vi "configureOutput.vi"(6 "sofwareTrigger?":bool, 8 "error in (no error)":errorcluster, 9 "Data":variant, 10 "Config":T1, 11 "SpinCore in":refnum<class "SpinCore.lvclass">) -> (0 "error out":errorcluster, 3 "SpinCore out":refnum<class "SpinCore.lvclass">)   [LabVIEW 2011, in "Hardware.lvlib" / "Channels.lvlib" / "SpinCore.lvclass"]
doc: "Data is a varient cluster. \n\nThe varient is transformed into the correct cluster, and that cluster is stored.\n(Not Implemented for Ramp function)"
uses:
  SpinCore.lvclass
  Generic/DDSOutput.lvclass
  SpinCore.lvclass/SpinCore.ctl
panel:
  out "Data":dbl
  out "load time":dbl
  out "data (time, freq, amplitude, phase)":dbl[][](array[numeric]) format="%#.7g"
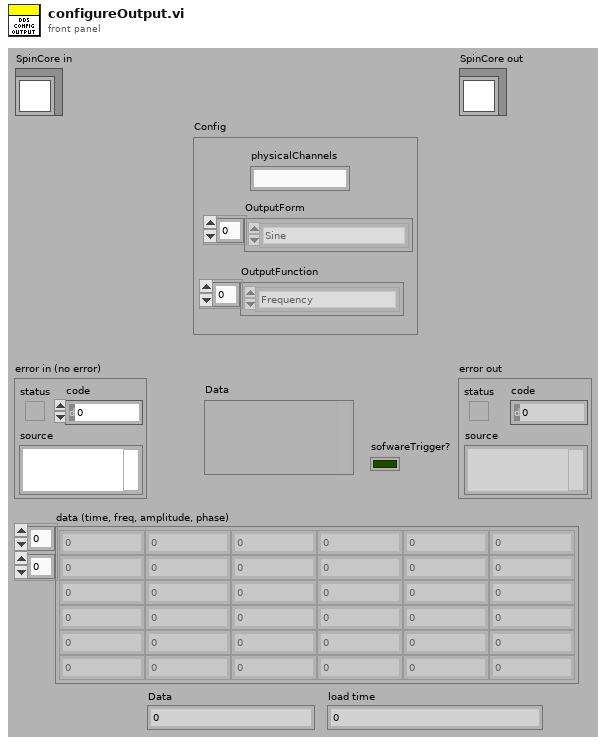
[diagram p1: front panel]
types:
  T1 = cluster{"OutputForm":enum16{"Sine", "Square", "Triangle", "Arbitrary"}[], "OutputFunction":enum16{"Frequency", "Ramp", "Sequence"}[], "physicalChannels":string}
  T2 = cluster{"Frequency(MHz)":dbl, "Amplitude":dbl, "Phase":dbl, "OutputForm":enum16{"Sine", "Square", "Triangle", "Arbitrary"}}[]
  T3 = cluster{"data (time, freq, amplitude, phase)":dbl[][]}
  T4 = cluster{"data (time, freq, amplitude, phase)":dbl[][]}[]
  T5 = cluster{"Frequency(MHz)":dbl, "Amplitude":dbl, "Phase":dbl, "OutputForm":enum16{"Sine", "Square", "Triangle", "Arbitrary"}}
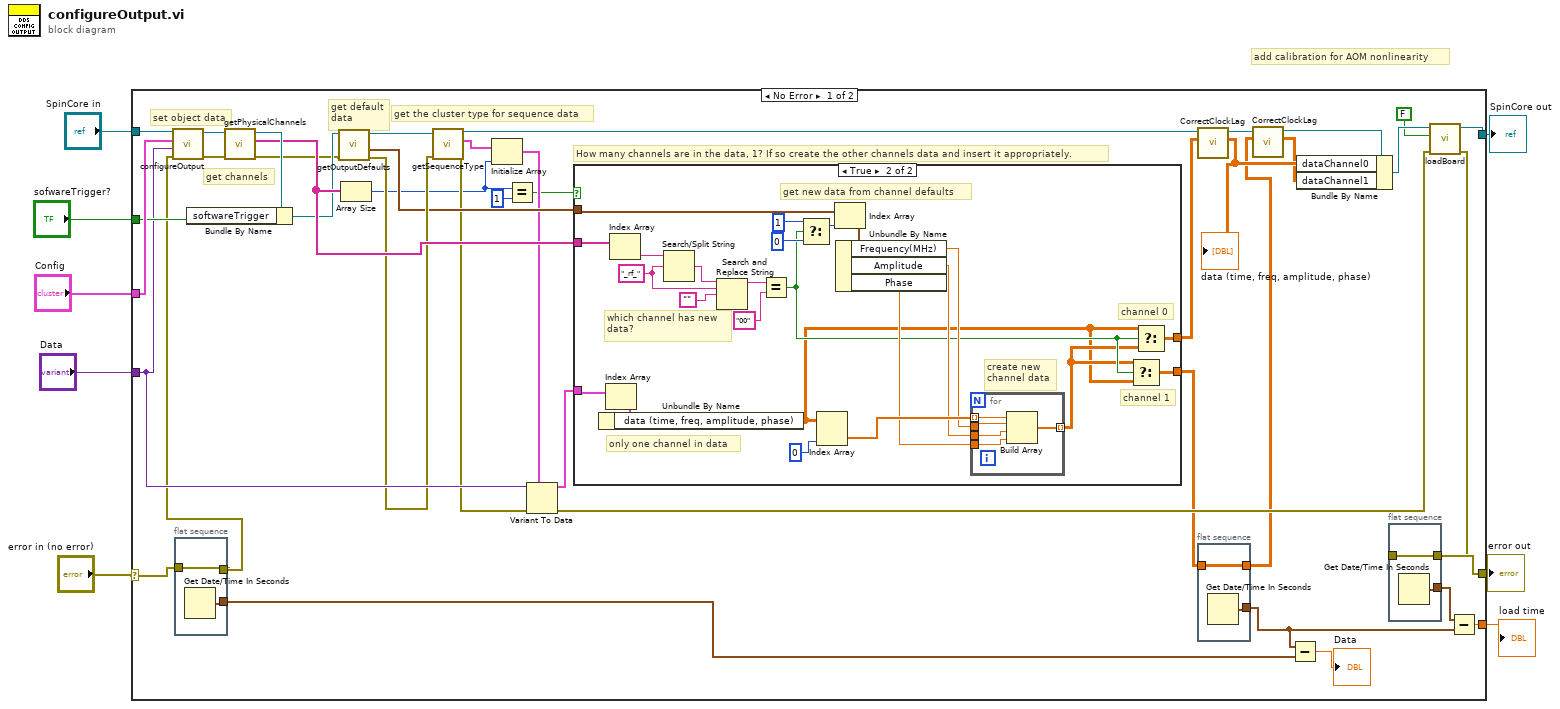
[diagram p0: block diagram]
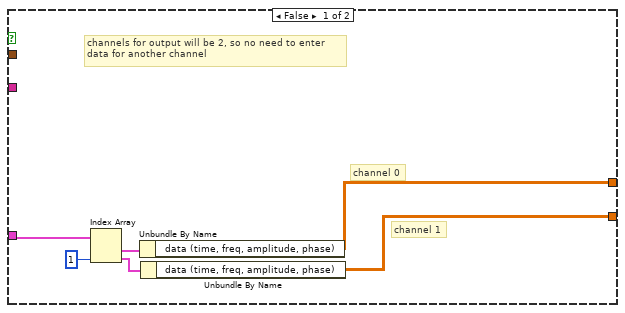
[diagram p2: hidden frame]
diagram:
  # "add calibration for AOM nonlinearity"
  n1 = case shown="No Error" "error in (no error)" {
    selector: "error in (no error)" -> [w22 w91]
    tunnel: [w26 w91] -> w8
    tunnel: [w46 w92] -> w7
    tunnel: "SpinCore in" -> [w49 w92]
    tunnel: "Config" -> [w48 _]
    tunnel: "Data" -> [w40 _]
    tunnel: "sofwareTrigger?" -> [w45 _]
    tunnel: [w23 _] -> w1
    frame No Error {
      # "get default\ndata"
      # "get channels"
      # "set object data"
      # "get the cluster type for sequence data"
      # "How many channels are in the data, 1? If so create the other channels data and insert it appropriately."
      n2 = call-parent "configureOutput.vi"("error in (no error)"=w21, "Data"=w40, "Config"=w48, "DDSOutput in"=w49) -> ("error out"=w44:errorcluster, "DDSOutput out"=w43:refnum<class "SpinCore.lvclass">)  [unwired: 6 in]
      n3 = flat-sequence {
        tunnel: [w51] -> w21
        tunnel: w22 -> [w51]
        tunnel: [w50] -> w17
        frame #0 {
          n4 = Get Date/Time In Seconds() -> (seconds since 1Jan1904=w50:timestamp)
        }
      }
      n5 = call "getPhysicalChannels.vi"("error in (no error)"=w44, "DDSOutput in"=w43) -> ("error out"=w36:errorcluster, "physicalChannels"=w41:string[], "DDSOutput out"=w42:refnum<class "SpinCore.lvclass">)  [unwired: 7 in]
      n6 = Bundle By Name(cluster=w42, "softwareTrigger"=w45) -> (w37:refnum<class "SpinCore.lvclass">)
      n7 = call "getOutputDefaults.vi"("error in (no error)"=w36, "DDSOutput in"=w37) -> ("error out"=w35:errorcluster, "Defaults"=w34:T2, "DDSOutput out"=w38:refnum<class "SpinCore.lvclass">)  [unwired: 6 in, 1 out]
      n8 = Array Size(array=w41) -> (size(s)=w29:i32)
      n9 = call "getSequenceType.vi"("error in (no error)"=w35, "DDSOutput in"=w38) -> ("error out"=w32:errorcluster, "Sequence"=w33:T3, "DDSOutput out"=w15:refnum<class "SpinCore.lvclass">)  [unwired: 7 in]
      n10 = Initialize Array(w33, w29) -> (w31:T4)
      n11 = Equal?(x=w29, y=1) -> (x = y?=w28:bool)
      n12 = Variant To Data(error in=w32, type=w31, Variant=w40) -> (data=w30:T4, error out=w20:errorcluster)
      n13 = case shown="True" w28 {
        tunnel: w41 -> [_ w81]
        tunnel: w34 -> [_ w74]
        tunnel: w30 -> [w61 w75]
        tunnel: [w59 w65] -> w14
        tunnel: [w57 w64] -> w19
        frame False {
          # "channel 1"
          # "channel 0"
          # "channels for output will be 2, so no need to enter\ndata for another channel"
          n14 = Index Array(array=w61, index #2=1) -> (element #1=w60:T3, element #2=w58:T3)  [unwired: 1 in]
          n15 = Unbundle By Name(w60) -> ("data (time, freq, amplitude, phase)"=w59:dbl[][])
          n16 = Unbundle By Name(w58) -> ("data (time, freq, amplitude, phase)"=w57:dbl[][])
        }
        frame True {
          w83 = "_rf_"
          # "get new data from channel defaults"
          # "only one channel in data"
          # "create new\nchannel data"
          # "channel 1"
          # "channel 0"
          # "which channel has new\ndata?"
          n17 = Index Array(array=w75) -> (element=w73:T3)  [unwired: 1 in]
          n18 = Unbundle By Name(w73) -> ("data (time, freq, amplitude, phase)"=w62:dbl[][])
          n19 = Index Array(array=w81) -> (element=w85:string)  [unwired: 1 in]
          n20 = Search/Split String(string=w85, search string/char (-)=w83) -> (match + rest of string=w84:string)  [unwired: 1 in, 2 out]
          n21 = Search and Replace String(input string=w84, search string=w83, replace string="") -> (result string=w79:string)  [unwired: 5 in, 3 out]
          n22 = Equal?(x=w79, y="00") -> (x = y?=w66:bool)
          n23 = Select(t=1, s=w66, f=0) -> (s? t:f=w78:i32)
          n24 = Index Array(array=w62, index (col)=0) -> (element=w70:dbl[])  [unwired: 1 in]
          n25 = Index Array(array=w74, index=w78) -> (element=w72:T5)
          n26 = Unbundle By Name(w72) -> ("Frequency(MHz)"=w69:dbl, "Amplitude"=w68:dbl, "Phase"=w67:dbl)
          n27 = for {
            tunnel: w70 -> [w90] mode=indexing
            tunnel: w69 -> [w89]
            tunnel: w68 -> [w88]
            tunnel: w67 -> [w87]
            tunnel: [w86] -> w63 mode=indexing
            n28 = Build Array(w90, w89, w88, w87) -> (w86:dbl[])
          }
          n29 = Select(t=w63, s=w66, f=w62) -> (s? t:f=w64:dbl[][])
          n30 = Select(t=w62, s=w66, f=w63) -> (s? t:f=w65:dbl[][])
        }
      }
      n31 = call "CorrectClockLag.vi"("data (time, freq, amplitude, phase)"=w14, "SpinCore in"=w15) -> ("data (time, freq, amplitude, phase)"=w13:dbl[][], "SpinCore out"=w12:refnum<class "SpinCore.lvclass">)  [unwired: 7 in, 1 out]
      "data (time, freq, amplitude, phase)" <- w13
      n32 = flat-sequence {
        tunnel: [w55] -> w18
        tunnel: [w54] -> w10
        tunnel: w19 -> [w54]
        frame #0 {
          n33 = Get Date/Time In Seconds() -> (seconds since 1Jan1904=w55:timestamp)
        }
      }
      n34 = call "CorrectClockLag.vi"("data (time, freq, amplitude, phase)"=w10, "SpinCore in"=w12) -> ("data (time, freq, amplitude, phase)"=w11:dbl[][], "SpinCore out"=w9:refnum<class "SpinCore.lvclass">)  [unwired: 7 in, 1 out]
      n35 = Subtract(x=w18, y=w17) -> (x-y=→"Data":dbl)
      n36 = Bundle By Name(cluster=w9, "dataChannel0"=w13, "dataChannel1"=w11) -> (w47:refnum<class "SpinCore.lvclass">)
      n37 = flat-sequence {
        tunnel: [w53] -> w24
        tunnel: [w52] -> w26
        tunnel: w25 -> [w52]
        frame #0 {
          n38 = Get Date/Time In Seconds() -> (seconds since 1Jan1904=w53:timestamp)
        }
      }
      n39 = call "loadBoard.vi"("error in (no error)"=w20, "continuous"=FALSE, "SpinCore in"=w47) -> ("error out"=w25:errorcluster, "SpinCore out"=w46:refnum<class "SpinCore.lvclass">)  [unwired: 7 in]
      n40 = Subtract(x=w24, y=w18) -> (x-y=w23:dbl)
    }
    frame Error {
    }
  }
  "error out" <- w8
  "SpinCore out" <- w7
  "load time" <- w1
